vi "Trigger.vi"(8 "Error In":errorcluster, 11 "object in":refnum<class "ByValue1.lvclass">) -> (0 "Error Out":errorcluster, 3 "object out":refnum<class "ByValue1.lvclass">)   [LabVIEW 2020, in "ByValue1.lvclass"]
doc: "This method gets called every time the trigger elaps"
uses:
  ByValue1.lvclass
  ByValue1.lvclass/ByValue1.ctl
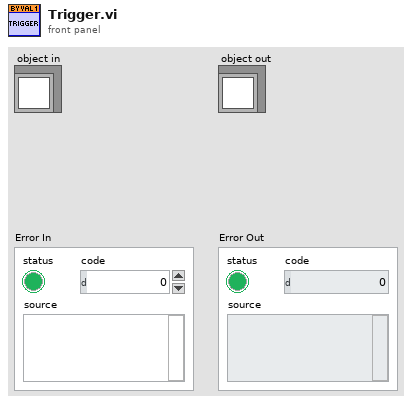
[diagram p1: front panel]
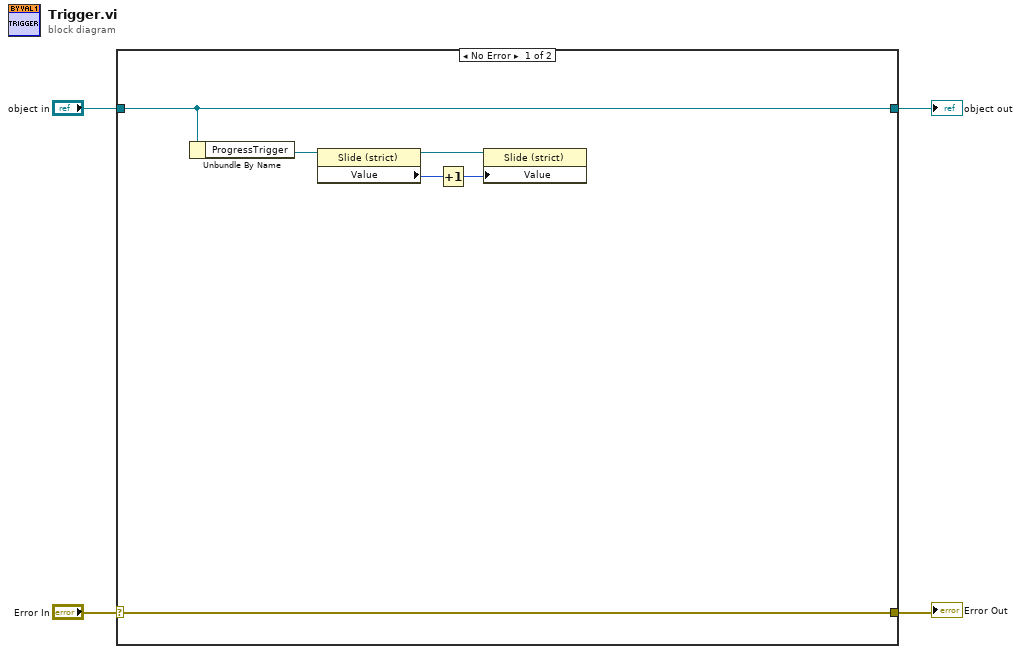
[diagram p0: block diagram]
diagram:
  n1 = case shown="No Error" "Error In" {
    selector: "Error In" -> [w10 w12]
    tunnel: [w10 w12] -> w3
    tunnel: [w9 w11] -> w1
    tunnel: "object in" -> [w9 w11]
    frame No Error {
      n2 = Unbundle By Name(w9) -> ("ProgressTrigger"=w8:refnum<vi>)
      n3 = property class="Slide (strict)"(reference=w8) -> (reference out=w7:refnum<vi>, "Value"=w6:u8)  [unwired: 1 in, 1 out]
      n4 = Increment(x=w6) -> (x+1=w5:u8)
      n5 = property class="Slide (strict)"(reference=w7, "Value"=w5) -> ()  [unwired: 1 in, 2 out]
    }
    frame Error {
    }
  }
  "Error Out" <- w3
  "object out" <- w1
